vi "gentec-M-Link.Query Cal Lambda.vi"(0 "VISA resource In":refnum<visa-resource-name>, 5 "error in (no error)":errorcluster) -> (11 "Data Read":string, 13 "Read Timeout":bool, 14 "VISA resource Out":refnum<visa-resource-name>, 16 "Cal Lambda":i32, 19 "error out":errorcluster)   [LabVIEW 2014, in "gentec-M-Link - Driver.lvlib"]
doc: "Data to write: pwv"
uses:
  gentec-M-Link - Driver.lvlib
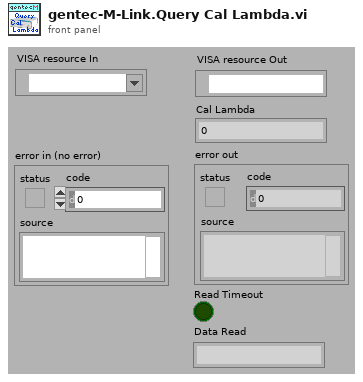
[diagram p1: front panel]
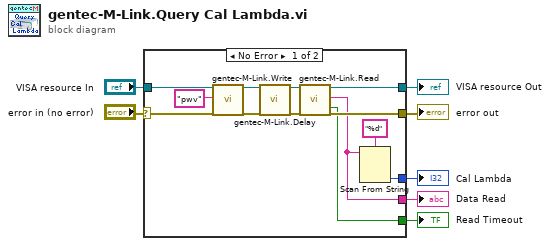
[diagram p0: block diagram]
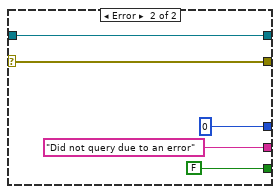
[diagram p2: hidden frame]
diagram:
  n1 = case shown="No Error" "error in (no error)" {
    selector: "error in (no error)" -> [w13 w25]
    tunnel: [w15 w25] -> w6
    tunnel: "VISA resource In" -> [w12 w24]
    tunnel: [w11 0] -> w4
    tunnel: [w10 w24] -> w3
    tunnel: [w9 FALSE ("Read Timeout")] -> w2
    tunnel: [w8 "Did not query due to an error" ("Data Read")] -> w1
    frame No Error {
      n2 = call "gentec-M-Link.Write.vi"("VISA resource (In)"=w12, "Data To Write"="pwv", "error in (no error)"=w13) -> ("VISA resource (Out)"=w18:refnum<visa-resource-name>, "error out"=w19:errorcluster)  [unwired: 14 in, 1 out]
      n3 = call "gentec-M-Link.Delay.vi"("VISA resource In"=w18, "error in (no error)"=w19) -> ("VISA resource Out"=w17:refnum<visa-resource-name>, "error out"=w16:errorcluster)  [unwired: 16 in]
      n4 = call "gentec-M-Link.Read.vi"("VISA resource (In)"=w17, "error in (no error)"=w16) -> ("VISA resource (Out)"=w10:refnum<visa-resource-name>, "Data Read"=w8:string, "Read Timeout"=w9:bool, "error out"=w15:errorcluster)  [unwired: 13 in, 1 out]
      n5 = Scan From String(format string="%d", input string=w8) -> (output 1=w11:i32)  [unwired: 3 in, 3 out]
    }
    frame Error {
    }
  }
  "error out" <- w6
  "Cal Lambda" <- w4
  "VISA resource Out" <- w3
  "Read Timeout" <- w2
  "Data Read" <- w1
